vi "ToFTestertester.vi"(8 "error in":errorcluster, 9 "I2C Channel":u8=1, 11 "ToFs":T1[](array[typedef])=[enum."ToF1", enum."ToF2", enum."ToF3", enum."ToF5"]) -> (0 "error out":errorcluster, 1 "ToF Online":bool[](array[boolean]), 2 "ToF Details":T2[](array[typedef]) {"I2C Slave Address" format="%02x"})   [LabVIEW 2017]
uses:
  Sensors/Time of Flight - VL6180/VL6180 Resource.ctl
  Type Defs/Relays.ctl
panel:
  out "count":u8
  in  "wait (ms)":u32=150
  in  "Attempts":i32=2
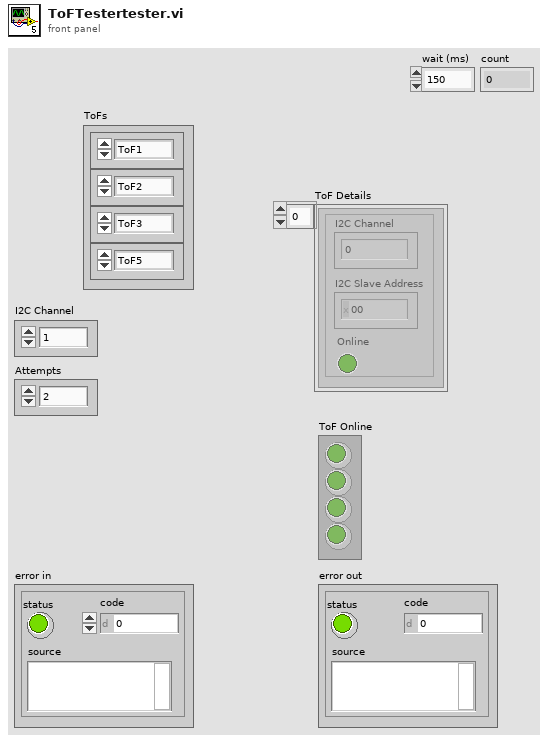
[diagram p1: front panel]
types:
  T1 = typedef "Relays.ctl" = enum16{"ToF1", "ToF2", "ToF3", "ToF4", "ToF5", "ToF6", "ToF7", "ToF8", "SensePwr", "All"}
  T2 = typedef "VL6180 Resource.ctl" = cluster{"I2C Channel":u8, "I2C Slave Address":u8, "Online":bool}
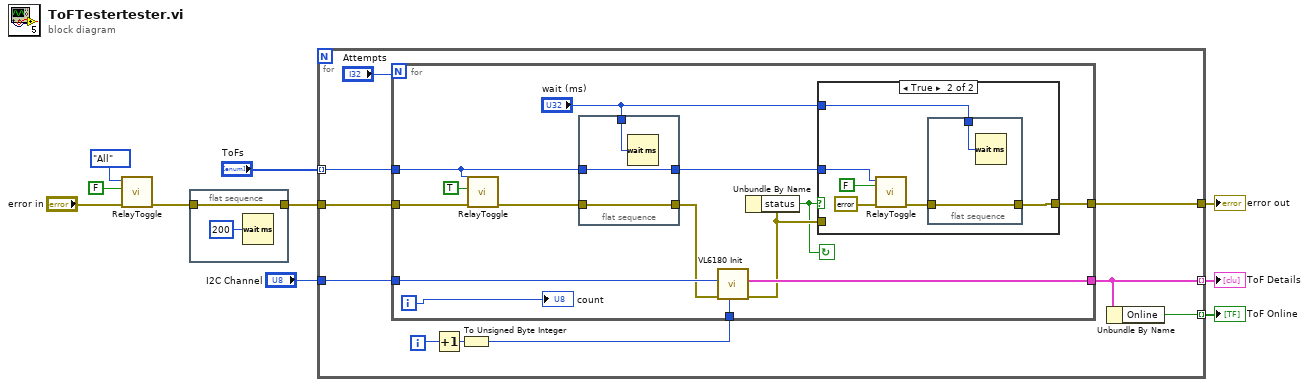
[diagram p0: block diagram]
diagram:
  n1 = call "RelayToggle.vi"("error in"="error in", "Power"=FALSE, "Relay"=Relays."All") -> ("error out"=w2:errorcluster)  [unwired: 8 in]
  n2 = flat-sequence {
    tunnel: w2 -> [w12]
    tunnel: [w12] -> w1
    frame #0 {
      n3 = Wait (ms)(milliseconds to wait=u32 200) -> ()  [unwired: 1 out]
    }
  }
  n4 = for {
    tunnel: w1 -> [w22]
    tunnel: "I2C Channel" -> [w20]
    tunnel: [w14] -> w9
    tunnel: [w16] -> w8 mode=indexing
    tunnel: [w15] -> w7 mode=indexing
    tunnel: "ToFs" -> [w13] mode=indexing
    i -> [w21]
    n5 = Increment(x=w21) -> (x+1=w19:i32)
    n6 = To Unsigned Byte Integer(number=w19) -> (unsigned 8bit integer=w18:u8)
    n7 = for {
      N: "Attempts" -> [_]
      tunnel: w22 -> [w27]
      tunnel: w20 -> [w36]
      tunnel: w18 -> [w34]
      tunnel: [w33] -> w14
      tunnel: [w32] -> w16
      tunnel: w13 -> [w24]
      i -> [w30]
      stop <- w28 continue-if-true
      n8 = call "RelayToggle.vi"("error in"=w27, "Power"=TRUE, "Relay"=w24) -> ("error out"=w26:errorcluster)  [unwired: 8 in]
      n9 = flat-sequence {
        tunnel: [w48] -> w35
        tunnel: w26 -> [w48]
        tunnel: "wait (ms)" -> [w47]
        tunnel: w24 -> [w46]
        tunnel: [w46] -> w23
        frame #0 {
          n10 = Wait (ms)(milliseconds to wait=w47) -> ()  [unwired: 1 out]
        }
      }
      n11 = call "VL6180 Init.vi"("Change Slave Address"=w34, "Error In"=w35, "I2C Channel"=w36) -> ("Error Out"=w29:errorcluster, "VL6180 Resource"=w32:T2)  [unwired: 6 in, 1 out]
      n12 = Unbundle By Name(w29) -> ("status"=w28:bool)
      n13 = case shown="True" w28 {
        tunnel: [w37 w40] -> w33
        tunnel: "wait (ms)" -> [_ w43]
        tunnel: w29 -> [w37 _]
        tunnel: w23 -> [_ w38]
        frame False {
        }
        frame True {
          n14 = call "RelayToggle.vi"("error in"=errorcluster {"status"=FALSE, "code"=0, "source"=""} ("error in (no error)"), "Power"=FALSE, "Relay"=w38) -> ("error out"=w39:errorcluster)  [unwired: 8 in]
          n15 = flat-sequence {
            tunnel: w43 -> [w45]
            tunnel: [w44] -> w40
            tunnel: w39 -> [w44]
            frame #0 {
              n16 = Wait (ms)(milliseconds to wait=w45) -> ()  [unwired: 1 out]
            }
          }
        }
      }
      "count" <- w30
    }
    n17 = Unbundle By Name(w16) -> ("Online"=w15:bool)
  }
  "error out" <- w9
  "ToF Details" <- w8
  "ToF Online" <- w7
